vi "updateRate.vi"(8 "error in (no error)":errorcluster, 11 "Model in":refnum<class "Model.lvclass">) -> (0 "error out":errorcluster, 3 "Model out":refnum<class "Model.lvclass">)   [LabVIEW 2015]
uses:
  <userlib>/Common/ILC/ILC/ILC.lvclass
  Model.lvclass
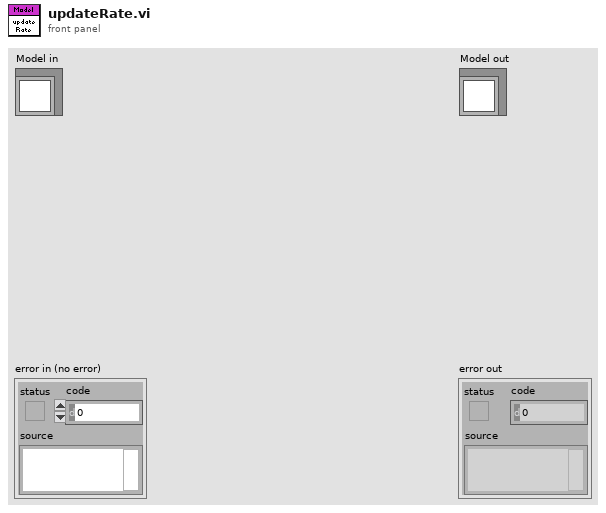
[diagram p1: front panel]
types:
  T1 = typedef "ILCCommon.lvlib/ILCTypedefs.lvlib/ADC Settings.ctl" = cluster{"Input Channels":T2, "Scan Rate (Hz) ":T3, "PGA Gain Coefficient":u8}
  T2 = typedef "ILCCommon.lvlib/ILCConfiguration.lvlib/Input Channels.ctl" = enum16{"Channel 0", "3 Channels", "5 Channels"}
  T3 = typedef "ILCCommon.lvlib/ILCConfiguration.lvlib/Scan Rates.ctl" = enum16{"50", "60", "100", "120", "200", "240", "300", "400", "480", "600", "1200", "2400", "4800"}
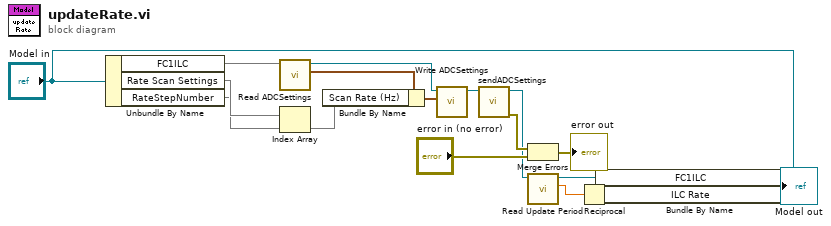
[diagram p0: block diagram]
diagram:
  n1 = Unbundle By Name("Model in") -> ("FC1ILC"=w15, "Rate Scan Settings"=w17, "RateStepNumber"=w16)
  n2 = call <userlib>:"Read ADCSettings.vi"("ILC in"=w15) -> ("ADC Settings"=w14:T1, "ILC out"=w13:refnum<class "ILC.lvclass">)  [unwired: 9 in]
  n3 = Index Array(array=w17, index=w16) -> (element=w11)
  n4 = Bundle By Name(cluster=w14, "Scan Rate (Hz)"=w11) -> (w12:T1)
  n5 = call <userlib>:"Write ADCSettings.vi"("ADC Settings"=w12, "ILC in"=w13) -> ("ILC out"=w8:refnum<class "ILC.lvclass">)  [unwired: 9 in]
  n6 = call <userlib>:"sendADCSettings.vi"("ILC in"=w8) -> ("error out"=w7:errorcluster, "ILC out"=w3:refnum<class "ILC.lvclass">)  [unwired: 9 in]
  n7 = Merge Errors(w7, "error in (no error)") -> (→"error out":errorcluster)
  n8 = call <userlib>:"Read Update Period.vi"("ILC in"=w3) -> ("Update Period"=w4:dbl[unit], "ILC out"=w2:refnum<class "ILC.lvclass">)  [unwired: 9 in]
  n9 = Reciprocal(x=w4) -> (1/x=w1:dbl[unit])
  n10 = Bundle By Name(cluster="Model in", "FC1ILC"=w2, "ILC Rate"=w1) -> (→"Model out":cluster{})
